vi "1D Polar to Rectangular PtByPt.vi"(2 "phase":dbl format="%0.2f", 3 "magnitude":dbl format="%0.2f") -> (0 "y":dbl format="%0.2f", 1 "x":dbl format="%0.2f")   [LabVIEW 2020, in "NI_PtbyPt.lvlib"]
doc: "Converts the polar representation of a complex number into the rectangular representation of the complex number."
uses:
  NI_PtbyPt.lvlib
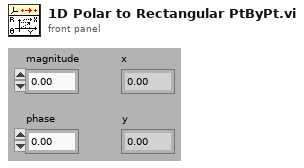
[diagram p1: front panel]
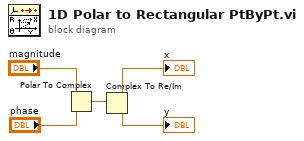
[diagram p0: block diagram]
diagram:
  n1 = Polar To Complex(1:"phase", 2:"magnitude") -> (0:w3:cdb)
  n2 = Complex To Re/Im(x + iy=w3) -> (x=→"x":dbl, y=→"y":dbl)
